vi "DATA_STREAM.vi"(10 "Payload":T1={"message_rate"=10, "stream_id"=0, "on_off"=FALSE}) -> (3 "MAVLink Message":u8[](array[numeric]))   [LabVIEW 2014]
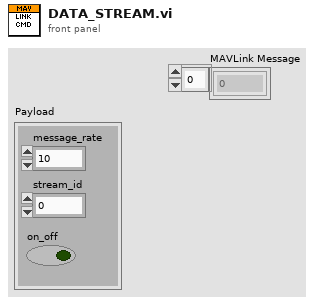
[diagram p1: front panel]
types:
  T1 = cluster{"message_rate":u16, "stream_id":u8, "on_off":bool}
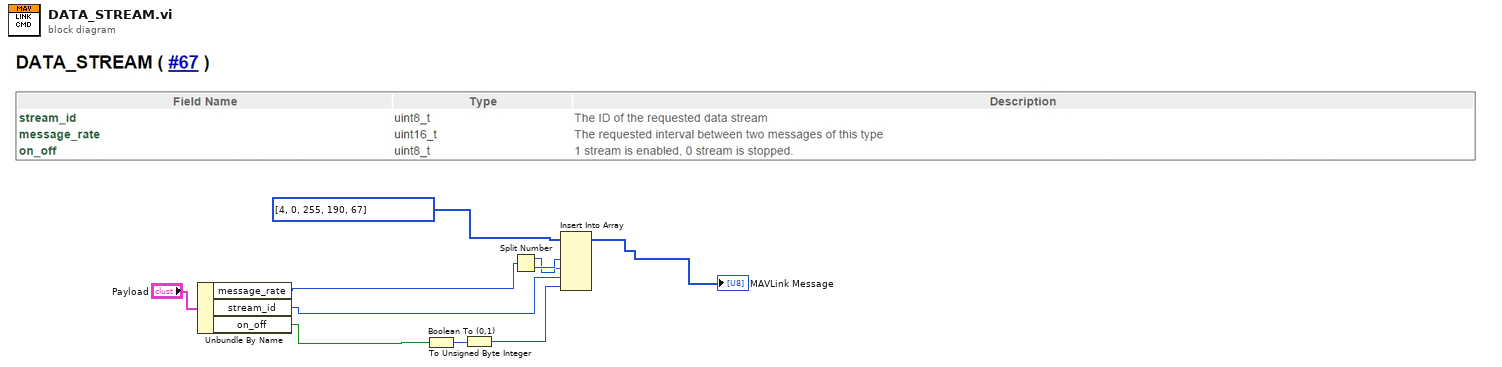
[diagram p0: block diagram]
diagram:
  n1 = Unbundle By Name("Payload") -> ("message_rate"=w7:u16, "stream_id"=w6:u8, "on_off"=w5:bool)
  n2 = Boolean To (0,1)(Boolean=w5) -> (0, 1=w10:i16)
  n3 = To Unsigned Byte Integer(number=w10) -> (unsigned 8bit integer=w9:u8)
  n4 = Split Number(x=w7) -> (hi(x)=w3:u8, lo(x)=w4:u8)
  n5 = Insert Into Array(array=u8[] [4, 0, 255, 190, 67], new element #1=w4, new element #2=w3, new element #3=w6, new element #4=w9) -> (→"MAVLink Message":u8[])  [unwired: 1 in]
